vi "1Darray_sum_ave_optic_sub.vi"(3 "1D array":dbl[](array[numeric])) -> (0 "Average":ext, 1 "Sum":ext)   [LabVIEW 2021]
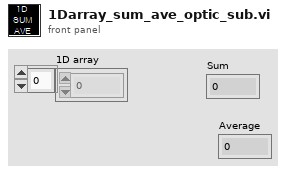
[diagram p1: front panel]
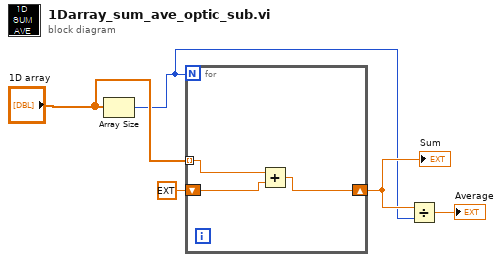
[diagram p0: block diagram]
diagram:
  n1 = Array Size(array="1D array") -> (size(s)=w2:i32)
  n2 = for {
    N: w2 -> [_]
    tunnel: "1D array" -> [w8] mode=indexing
    shift-right: [w7] -> w3
    shift-left: ext 0.0 -> [w6]
    n3 = Add(x=w8, y=w6) -> (x+y=w7:ext)
  }
  "Sum" <- w3
  n4 = Divide(x=w3, y=w2) -> (x/y=→"Average":ext)
